vi "Select E_M Range.vi"(6 "Data":string[][](array[string]), 7 "STD Select Ref.":refnum<vi>, 8 "에러 입력":errorcluster caption="에러 입력(에러 없음)", 11 "Func in":string) -> (0 "에러 출력":errorcluster, 2 "STD Select Value":string, 3 "Func out":string, 4 "STD Resolution":string[][](array[string]))   [LabVIEW 2020]
uses:
  Controls/Cmd_STD select.ctl
  Variables/Global_Cal STD.vi
  Public/Polymorph/Array Dedup_2D Str.vi
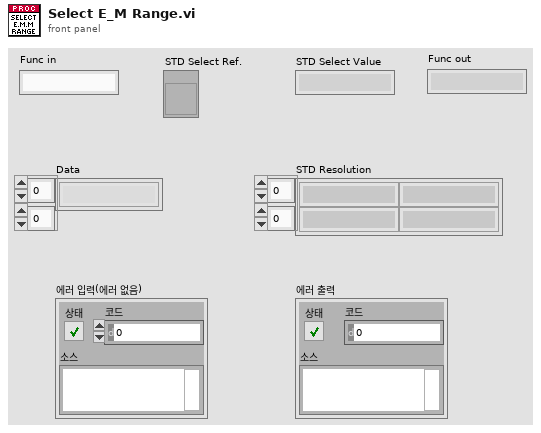
[diagram p1: front panel]
types:
  T1 = typedef "Cmd_STD select.ctl" = enum16{"기본", "DMM", "Electronic Micrometer", "Fine Angle Generator", "Measuring Projector", "Precision Square", "Power Supply", "Ring Gauge", "Straight Edge", "Thermo-Hygrometer", "Calibrator"}
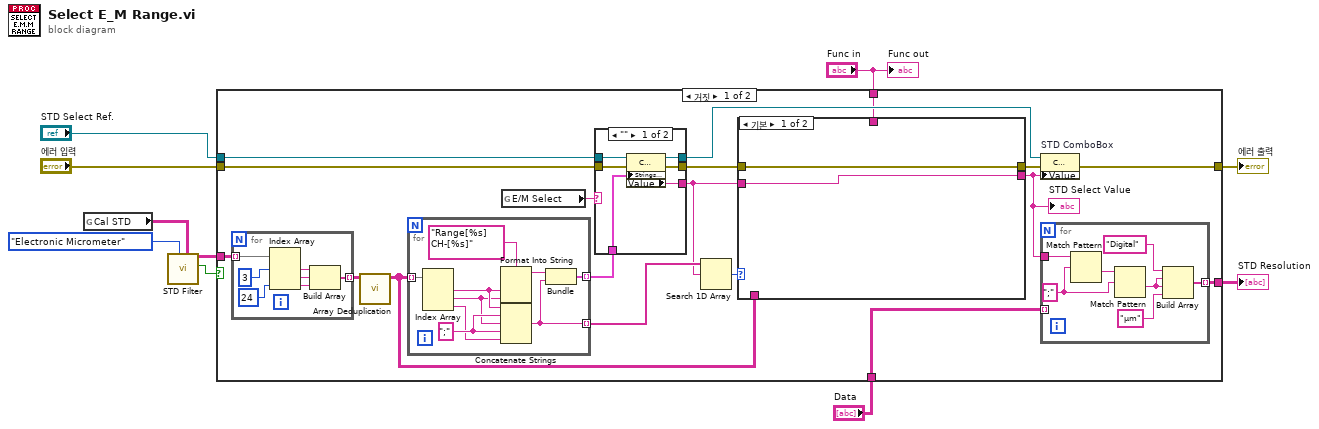
[diagram p0: block diagram]
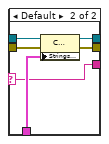
[diagram p2: hidden frame]
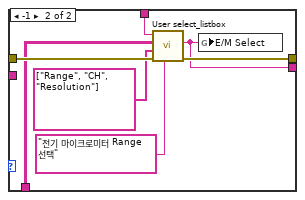
[diagram p3: hidden frame]
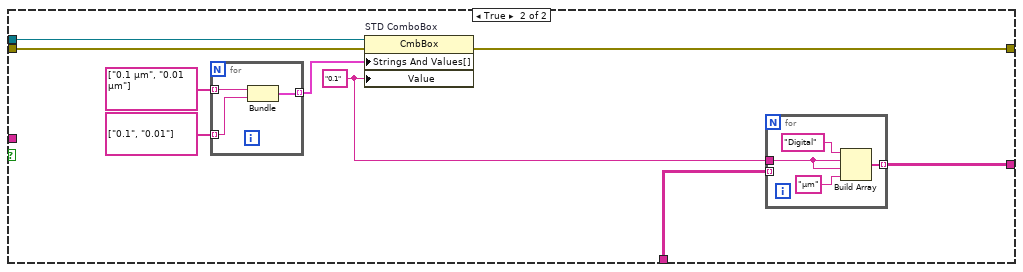
[diagram p4: hidden frame]
diagram:
  n1 = global read "Global_Cal STD.vi" "Cal STD"() -> (w3:string[][])
  n2 = call "STD Filter.vi"("Cal STD in"=w3, "STD select"=Cmd_STD_select."Electronic Micrometer") -> ("비어있음?"=w1:bool, "DATA 출력"=w2:string[][])  [unwired: 5 in, 3 out]
  n3 = case shown="거짓" w1 {
    tunnel: [w28 w79] -> w10
    tunnel: "에러 입력" -> [w27 w81]
    tunnel: w2 -> [w26 _]
    tunnel: "STD Select Ref." -> [w18 w80]
    tunnel: "Data" -> [w17 w74]
    tunnel: [w16 w73] -> w7
    tunnel: "Func in" -> [w14 _]
    frame False {
      n4 = for {
        tunnel: w26 -> [w56] mode=indexing
        tunnel: [w50] -> w25 mode=indexing
        n5 = Index Array(array=w56, index #1=3 ("비활성화된 인덱스 (열)"), index #3=24 ("인덱스 (열)")) -> (element #1=w52:string, element #2=w53:string, element #3=w51:string)  [unwired: 1 in]
        n6 = Build Array(w52, w53, w51) -> (w50:string[])
      }
      n7 = call-poly "Array Deduplication.vi"("배열 in"=w25) -> ("배열 out"=w23:string[][])  [unwired: 9 in, 1 out]
      n8 = for {
        tunnel: w23 -> [w72] mode=indexing
        tunnel: [w69] -> w24 mode=indexing
        tunnel: [w64] -> w15 mode=indexing
        w68 = ";" ("포맷 문자열")
        n9 = Index Array(array=w72) -> (element #1=w67:string, element #2=w66:string, element #3=w65:string)  [unwired: 3 in]
        n10 = Format Into String(format string="Range[%s] CH-[%s]" ("포맷 문자열"), w67, w66) -> (resulting string=w70:string)  [unwired: 2 in, 1 out]
        n11 = Concatenate Strings(w67, w68, w66, w68, w65) -> (w64:string)
        n12 = Bundle(w70, w64) -> (w69:cluster{string, string})  [unwired: 1 in]
      }
      n13 = global read "Global_Cal STD.vi" "E/M Select"() -> (w13:string)
      n14 = case shown="\"\"" w13 {
        selector: w13 -> [_ w35]
        tunnel: w27 -> [w34 w40]
        tunnel: w24 -> [w33 w39]
        tunnel: [w32 w38] -> w22
        tunnel: [w31 w37] -> w21
        tunnel: w18 -> [w30 w36]
        tunnel: [w29 w35] -> w12
        frame "" {
          n15 = property on="STD ComboBox" class="CmbBox"(reference=w30, error in=w34, "Strings And Values[]"=w33) -> (reference out=w31:refnum<vi>, error out=w32:errorcluster, "Value"=w29:string)
        }
        frame Default {
          n16 = property on="STD ComboBox" class="CmbBox"(reference=w36, error in=w40, "Strings And Values[]"=w39) -> (reference out=w37:refnum<vi>, error out=w38:errorcluster)
        }
      }
      n17 = Search 1D Array(1D array=w15, element=w12) -> (index of element=w11:i32)  [unwired: 1 in]
      n18 = case shown="기본" w11 {
        tunnel: w23 -> [_ w46]
        tunnel: w22 -> [w42 w49]
        tunnel: [w42 w48] -> w19
        tunnel: [w41 w43] -> w20
        tunnel: w12 -> [w41 _]
        tunnel: w14 -> [_ w45]
        frame Default {
        }
        frame -1 {
          n19 = call "User select_listbox.vi"("리스트명"="전기 마이크로미터 Range 선택", "error in"=w49, "Col Header in"=string[] ["Range", "CH", "Resolution"], "Data in"=w46, "Func in"=w45) -> ("error out"=w48:errorcluster, "Text out"=w43:string)  [unwired: 3 in, 2 out]
          n20 = global write "Global_Cal STD.vi" "E/M Select"(w43) -> ()
        }
      }
      "STD Select Value" <- w20
      n21 = property on="STD ComboBox" class="CmbBox"(reference=w21, error in=w19, "Value"=w20) -> (error out=w28:errorcluster)  [unwired: 1 out]
      n22 = for {
        tunnel: w20 -> [w58]
        tunnel: [w63] -> w16 mode=indexing
        tunnel: w17 -> [_] mode=indexing
        w59 = ";" ("정규식")
        n23 = Match Pattern(string=w58, regular expression=w59) -> (after substring=w60:string)  [unwired: 1 in, 3 out]
        n24 = Match Pattern(string=w60, regular expression=w59) -> (after substring=w57:string)  [unwired: 1 in, 3 out]
        n25 = Build Array("Digital" ("원소"), w57, w57, "μm" ("원소")) -> (w63:string[])
      }
    }
    frame True {
      w75 = "0.1" ("값")
      n26 = for {
        tunnel: string[] ["0.1 μm", "0.01 μm"] -> [w88] mode=indexing
        tunnel: string[] ["0.1", "0.01"] -> [w87] mode=indexing
        tunnel: [w86] -> w76 mode=indexing
        n27 = Bundle(w88, w87) -> (w86:cluster{string, string})  [unwired: 1 in]
      }
      n28 = property on="STD ComboBox" class="CmbBox"(reference=w80, error in=w81, "Strings And Values[]"=w76, "Value"=w75) -> (error out=w79:errorcluster)  [unwired: 1 out]
      n29 = for {
        tunnel: w75 -> [w82]
        tunnel: [w85] -> w73 mode=indexing
        tunnel: w74 -> [_] mode=indexing
        n30 = Build Array("Digital" ("원소"), w82, w82, "μm" ("원소")) -> (w85:string[])
      }
    }
  }
  "에러 출력" <- w10
  "STD Resolution" <- w7
  "Func out" <- "Func in"
